vi "Get All Certificates.vi"(8 "error in (no error)":errorcluster, 11 "store":string="My") -> (0 "error out":errorcluster, 3 "Certificates":string[](array[string]))   [LabVIEW 2020, in "CodeSignAPI.lvlib"]
uses:
  <vilib>/AppBuilder/CodeSignAPI/CodeSignAPI.lvlib
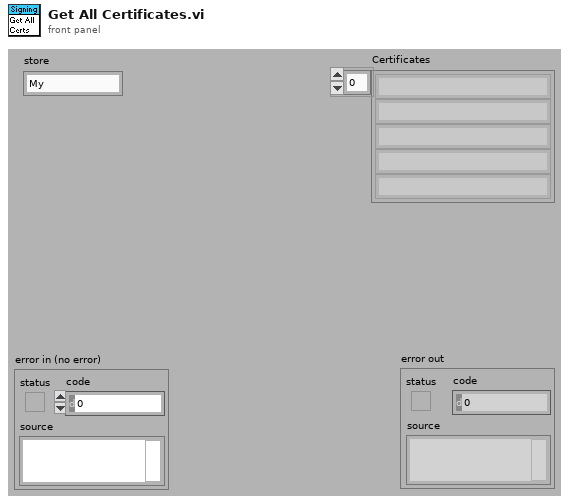
[diagram p1: front panel]
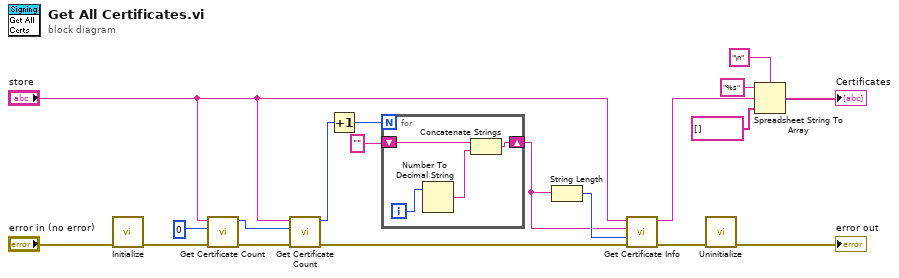
[diagram p0: block diagram]
diagram:
  n1 = call <vilib>:"Initialize.vi"("error in (no error)"="error in (no error)") -> ("error out"=w19:errorcluster)  [unwired: 10 out]
  n2 = call <vilib>:"Get Certificate Count.vi"("error in (no error)"=w19, "buffer size"=u32 0 ("bufsize"), "store"="store") -> ("error out"=w17:errorcluster, "count"=w14:u32)  [unwired: 1 in, 6 out]
  n3 = call <vilib>:"Get Certificate Count.vi"("error in (no error)"=w17, "buffer size"=w14, "store"="store") -> ("error out"=w16:errorcluster, "count"=w12:u32)  [unwired: 1 in, 6 out]
  n4 = Increment(x=w12) -> (x+1=w11:u32)
  n5 = for {
    N: w11 -> [_]
    shift-right: [w20] -> w8
    shift-left: "" -> [w21]
    i -> [w23]
    n6 = Number To Decimal String(number=w23) -> (decimal integer string=w22:string)  [unwired: 1 out]
    n7 = Concatenate Strings(w21, w22) -> (w20:string)
  }
  n8 = String Length(string=w8) -> (length=w9:i32)
  n9 = call <vilib>:"Get Certificate Info.vi"("error in (no error)"=w16, "bufsize"=w9, "buff"=w8, "store"="store") -> ("error out"=w15:errorcluster, "buff out"=w1:string)  [unwired: 1 in, 5 out]
  n10 = call <vilib>:"Uninitialize.vi"("error in (no error)"=w15) -> ("error out"=→"error out":errorcluster)  [unwired: 10 out]
  n11 = Spreadsheet String To Array(delimiter (Tab)="\n", format string="%s", spreadsheet string=w1, array type (2D Dbl)=string[] []) -> (array=→"Certificates":string[])
